vi "Monitor.vi"() -> ()   [LabVIEW 2015]
panel:
  out "TCP data out":string
  out "HTTP data out":string
  out "UDP data out":string
  out "Error Out 3":errorcluster
  out "Error Out 2":errorcluster
  out "Error Out":errorcluster
  out "Waveform Chart":i32[][](graph)
  in  "File Path Control":path=path "C:/Data/tcp_err.tdms"
  in  "milliseconds to wait":u32=60000
  in  "Stop Button":bool
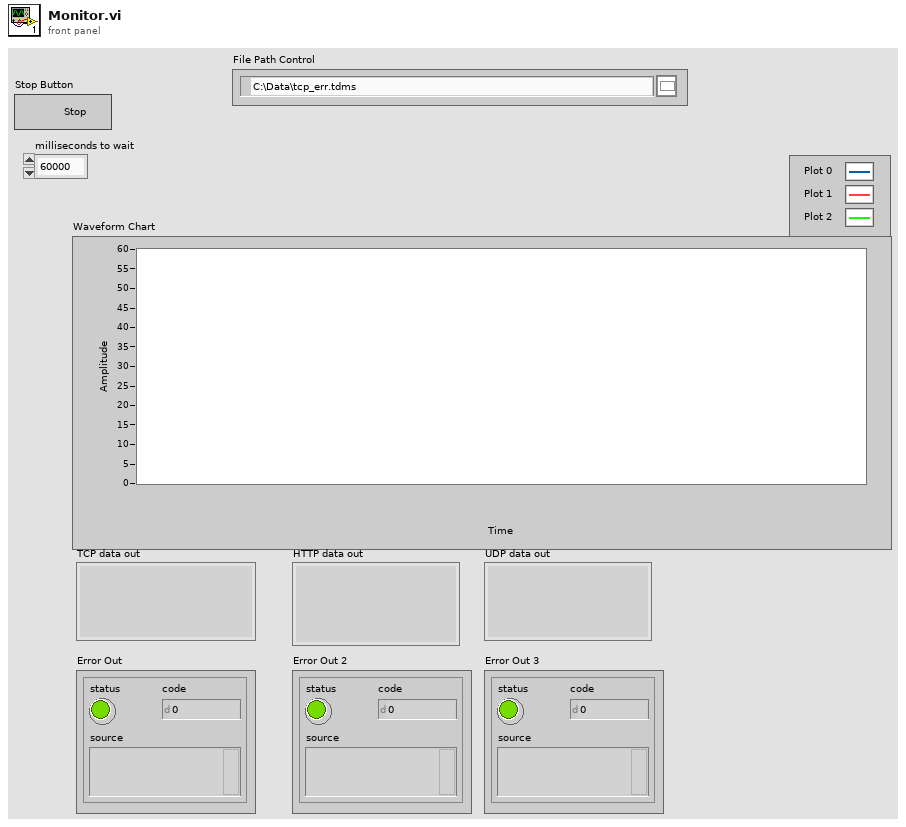
[diagram p1: front panel]
types:
  T1 = enum16{"open", "open or create", "create or replace", "create", "open (read-only)"}
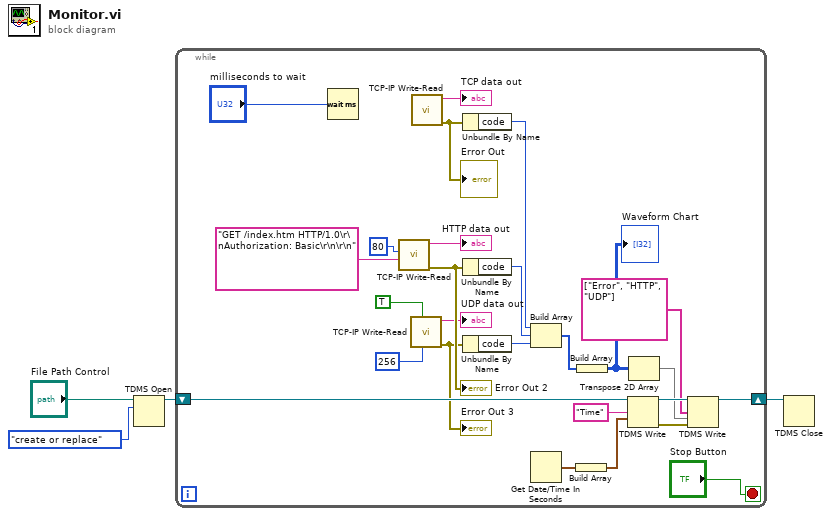
[diagram p0: block diagram]
diagram:
  n1 = TDMS Open(10:T1."create or replace" ("operation (0:open)"), 11:"File Path Control") -> (3:w2:refnum<k34>)  [unwired: 5 in, 1 out]
  n2 = while {
    shift-right: [w21] -> w1
    shift-left: w2 -> [w25]
    stop <- "Stop Button" stop-if-true
    n3 = Wait (ms)(milliseconds to wait="milliseconds to wait") -> ()  [unwired: 1 out]
    n4 = call "TCP-IP Write-Read.vi"("data in"="GET /index.htm HTTP/1.0\r\nAuthorization: Basic\r\n\r\n", "remote port or service name"=u16 80) -> ("Error Out"=w15:errorcluster, "data out"=→"HTTP data out":string)  [unwired: 8 in]
    "Error Out 2" <- w15
    n5 = call "TCP-IP Write-Read.vi"("bytes to read"=256, "UDP?"=TRUE) -> ("Error Out"=w11:errorcluster, "data out"=→"UDP data out":string)  [unwired: 8 in]
    "Error Out 3" <- w11
    n6 = call "TCP-IP Write-Read.vi"() -> ("Error Out"=w19:errorcluster, "data out"=→"TCP data out":string)  [unwired: 10 in]
    "Error Out" <- w19
    n7 = Unbundle By Name(w19) -> ("code"=w20:i32)
    n8 = Unbundle By Name(w15) -> ("code"=w14:i32)
    n9 = Unbundle By Name(w11) -> ("code"=w10:i32)
    n10 = Build Array(w20, w14, w10) -> (w16:i32[])
    n11 = Get Date/Time In Seconds() -> (seconds since 1Jan1904=w28:timestamp)
    n12 = Build Array(w28) -> (w27:timestamp[])
    n13 = Build Array(w16) -> (w13:i32[][])
    "Waveform Chart" <- w13
    n14 = TDMS Write(0:w25, 7:"Time", 9:w27) -> (4:w24:refnum<k34>, 15:w23:errorcluster)  [unwired: 3 in, 2 out]
    n15 = Transpose 2D Array(2D array=w13) -> (transposed array=w12:i32[][])
    n16 = TDMS Write(0:w24, 7:string[] ["Error", "HTTP", "UDP"], 9:w12, 11:w23) -> (4:w21:refnum<k34>)  [unwired: 2 in, 3 out]
  }
  n17 = TDMS Close(11:w1) -> ()  [unwired: 1 in, 2 out]
